vi "align label dialog.vi"() -> ()   [LabVIEW 2009]
uses:
  label position.ctl
panel:
  in  "label Position":T1
  in  "ACTION":bool
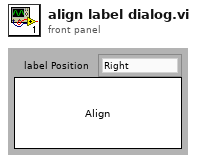
[diagram p1: front panel]
types:
  T1 = typedef "label position.ctl" = enum16{"Right", "Left", "Top left", "Top right"}
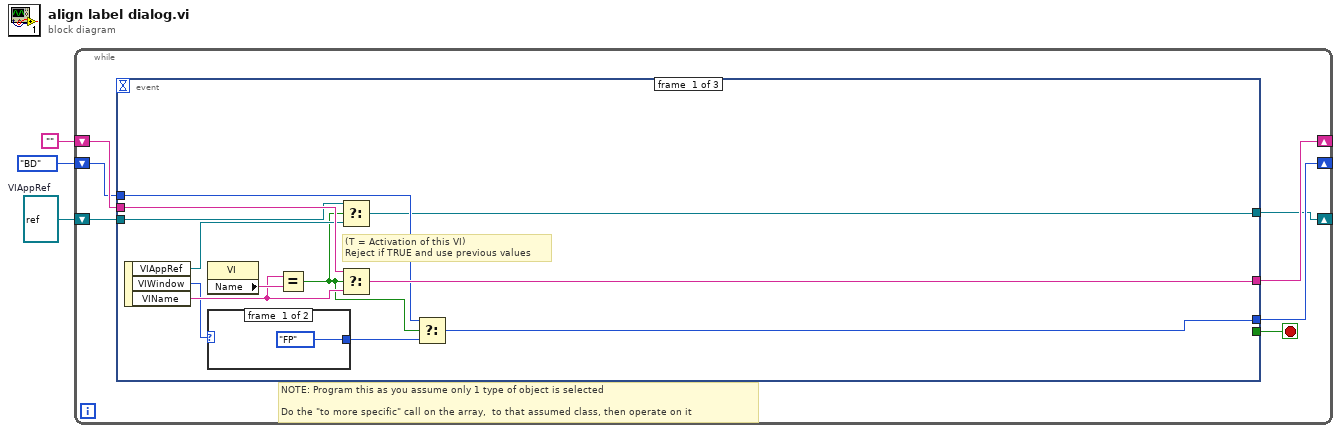
[diagram p0: block diagram]
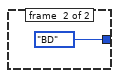
[diagram p2: hidden frame]
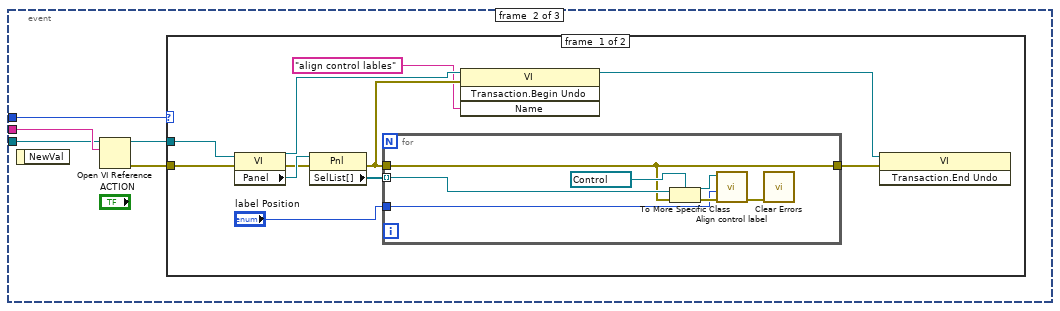
[diagram p3: hidden frame]
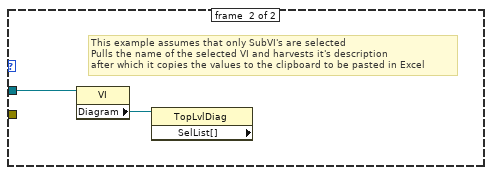
[diagram p4: hidden frame]
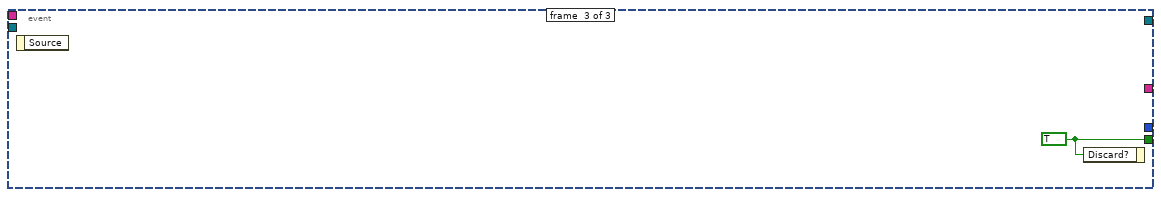
[diagram p5: hidden frame]
diagram:
  w1 = refnum<vi> refnum  # VIAppRef
  n1 = while {
    shift-right: [w10] -> _
    shift-left: "" -> [w9]
    shift-right: [w7] -> _
    shift-left: enum16{"FP", "BD"}."BD" -> [w6]
    shift-right: [w5] -> _
    shift-left: w1 -> [w4]
    stop <- w8 stop-if-true
    # "NOTE: Program this as you assume only 1 type of object is selected\n\nDo the \"to more specific\" call on the array,  to that assumed class, then operate on it"
    n2 = event shown="[1] \"ACTION\": Value Change" {
      selector: _ -> [_ _ _]
      dyn-events: _ -> [_ _ _]
      timeout: _ -> [_ _ _]
      tunnel: [w19 _ _] -> w10
      tunnel: w9 -> [w22 w29 _]
      tunnel: [_ _ w50] -> w8
      tunnel: [w17 _ _] -> w7
      tunnel: w6 -> [w18 w27 _]
      tunnel: [w13 _ _] -> w5
      tunnel: w4 -> [w12 w26 _]
      event #0 {
        # "(T = Activation of this VI)\nReject if TRUE and use previous values"
        n3 = event-data() -> ("VIAppRef"=w14:refnum<vi>, "VIWindow"=w16:i32, "VIName"=w20:string)  [unwired: 1 out]
        n4 = property class="VI"() -> ("Name"=w21:string)  [unwired: 2 in, 2 out]
        n5 = case shown="1" w16 {
          tunnel: [enum16{"FP", "BD"}."FP" enum16{"FP", "BD"}."BD"] -> w15
          frame #0 {
          }
          frame #1 {
          }
        }
        n6 = Equal?(x=w20, y=w21) -> (x = y?=w11:bool)
        n7 = Select(t=w12, s=w11, f=w14) -> (s? t:f=w13:refnum<vi>)
        n8 = Select(t=w22, s=w11, f=w20) -> (s? t:f=w19:string)
        n9 = Select(t=w18, s=w11, f=w15) -> (s? t:f=w17:enum16{"FP", "BD"})
      }
      event #1 {
        n10 = event-data() -> ()  [unwired: 2 out]
        n11 = Open VI Reference(application reference (local)=w26, vi path=w29) -> (vi reference=w28:refnum<vi>, error out=w25:errorcluster)  [unwired: 2 in, 2 out]
        n12 = case shown="\"FP\"" w27 {
          tunnel: w28 -> [w40 w49]
          tunnel: w25 -> [w35 _]
          frame #0 {
            n13 = property class="VI"(reference=w40, error in=w35) -> (reference out=w34:refnum<vi>, error out=w36:errorcluster, "Panel"=w39:refnum<vi>)
            n14 = property class="Pnl"(reference=w39, error in=w36) -> (error out=w32:errorcluster, "SelList[]"=w37:refnum<vi>[])  [unwired: 1 out]
            n15 = for {
              tunnel: "label Position" -> [w46]
              tunnel: w37 -> [w44] mode=indexing
              tunnel: w32 -> [w41]
              tunnel: [w41] -> w31
              n16 = To More Specific Class(target class=refnum<vi> refnum, reference=w44, error in=w41) -> (specific class reference=w43:refnum<vi>, error out=w47:errorcluster)
              n17 = call "Align control label.vi"("error in (no error)"=w47, "label Position"=w46, "Ctl Refnum"=w43) -> ("error out"=w42:errorcluster)  [unwired: 7 in, 1 out]
              n18 = call <vilib>:"Clear Errors.vi"("error in (no error)"=w42) -> ()  [unwired: 6 in, 1 out]
            }
            n19 = invoke class="VI" method="Transaction.Begin Undo"(reference=w34, error in=w32, "Name"="align control lables") -> (reference out=w33:refnum<vi>)  [unwired: 1 in, 3 out]
            n20 = invoke class="VI" method="Transaction.End Undo"(reference=w33, error in=w31) -> ()  [unwired: 1 in, 3 out]
          }
          frame #1 {
            # "This example assumes that only SubVI's are selected\nPulls the name of the selected VI and harvests it's description\nafter which it copies the values to the clipboard to be pasted in Excel"
            n21 = property class="VI"(reference=w49) -> ("Diagram"=w48:refnum<vi>)  [unwired: 1 in, 2 out]
            n22 = property class="TopLvlDiag" props=["SelList[]"](reference=w48) -> ()  [unwired: 1 in, 3 out]
          }
        }
      }
      event #2 {
        w50 = TRUE ("Discard?")
        n23 = event-data() -> ()  [unwired: 2 out]
        n24 = event-data("Discard?"=w50) -> ()  [unwired: 1 in, 1 out]
      }
    }
  }
